vi "Write DefaultAlternateCellBGKColor.vi"(8 "error in (no error)":errorcluster, 10 "CellBGKColorAlternate":u32(colorbox)=15790320, 11 "DataGridView in":refnum<class "DataGridView.lvclass">) -> (0 "error out":errorcluster, 3 "DataGridView out":refnum<class "DataGridView.lvclass">)   [LabVIEW 2014, in "DataGrid.lvlib" / "DataGridView.lvclass"]
uses:
  DataGridView.lvclass
  System.Drawing
  DataGridView.lvclass/DataGridView.ctl
  System.Windows.Forms
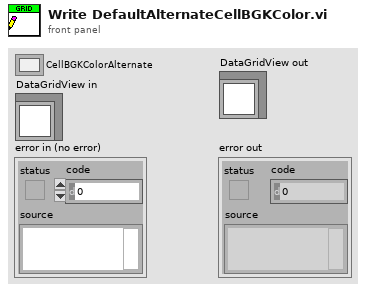
[diagram p1: front panel]
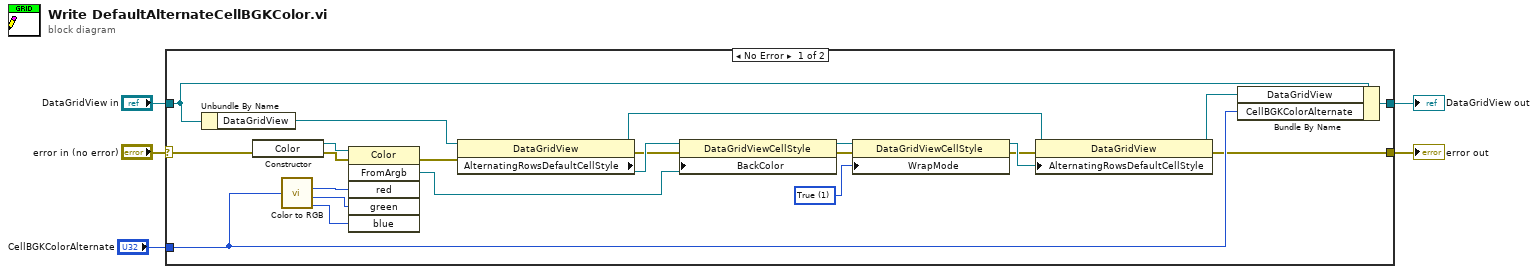
[diagram p0: block diagram]
diagram:
  n1 = case shown="No Error" "error in (no error)" {
    selector: "error in (no error)" -> [w19 w28]
    tunnel: [w12 w28] -> w4
    tunnel: [w27 w29] -> w2
    tunnel: "DataGridView in" -> [w21 w29]
    tunnel: "CellBGKColorAlternate" -> [w18 _]
    frame No Error {
      w10 = 1 items=["NotSet", "True", "False"] ("WrapMode")
      n2 = Unbundle By Name(w21) -> ("DataGridView"=w20:refnum<k24>)
      n3 = constructor class="Color"(error in=w19) -> (reference out=w22:refnum<k24>, error out=w23:errorcluster)  [unwired: 2 in, 1 out]
      n4 = call <vilib>:"Color to RGB.vi"("Color"=w18) -> ("R"=w24:u8, "G"=w25:u8, "B"=w26:u8)  [unwired: 1 out]
      n5 = invoke class="Color" method="FromArgb"(reference=w22, error in=w23, "red"=w24, "green"=w25, "blue"=w26) -> (error out=w14:errorcluster, "FromArgb"=w17:refnum<k24>)  [unwired: 1 in, 4 out]
      n6 = property class="DataGridView"(reference=w20, error in=w14) -> (reference out=w13:refnum<k24>, error out=w15:errorcluster, "AlternatingRowsDefaultCellStyle"=w16:refnum<k24>)
      n7 = property class="DataGridViewCellStyle"(reference=w16, error in=w15, "BackColor"=w17) -> (reference out=w9:refnum<k24>, error out=w8:errorcluster)
      n8 = property class="DataGridViewCellStyle"(reference=w9, error in=w8, "WrapMode"=w10) -> (reference out=w7:refnum<k24>, error out=w6:errorcluster)
      n9 = property class="DataGridView"(reference=w13, error in=w6, "AlternatingRowsDefaultCellStyle"=w7) -> (reference out=w11:refnum<k24>, error out=w12:errorcluster)
      n10 = Bundle By Name(cluster=w21, "DataGridView"=w11, "CellBGKColorAlternate"=w18) -> (w27:refnum<class "DataGridView.lvclass">)
    }
    frame Error {
    }
  }
  "error out" <- w4
  "DataGridView out" <- w2
